vi "PWM to Set.vi"(10 "Travel High Time":u32, 11 "Elevation High Time":u32) -> (2 "Travel Setpoint":dbl, 3 "Elevation Setpoint":dbl)   [LabVIEW 2011]
uses:
  MyGlobal.vi
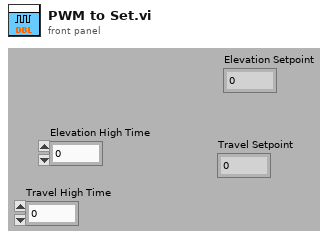
[diagram p1: front panel]
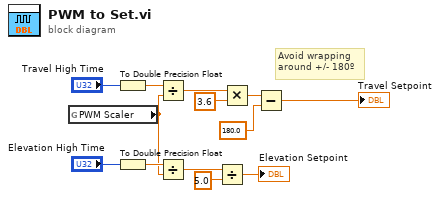
[diagram p0: block diagram]
diagram:
  # "Avoid wrapping\naround +/- 180º"
  n1 = global read "MyGlobal.vi" "PWM Scaler"() -> (w2:dbl)
  n2 = To Double Precision Float(number="Travel High Time") -> (double precision float=w8:dbl)
  n3 = To Double Precision Float(number="Elevation High Time") -> (double precision float=w11:dbl)
  n4 = Divide(x=w8, y=w2) -> (x/y=w4:dbl)
  n5 = Divide(x=w11, y=w2) -> (x/y=w3:dbl)
  n6 = Divide(x=w3, y=5.0) -> (x/y=→"Elevation Setpoint":dbl)
  n7 = Multiply(x=w4, y=3.6) -> (x*y=w6:dbl)
  n8 = Subtract(x=w6, y=180.0) -> (x-y=→"Travel Setpoint":dbl)
